vi "DropDown VI Wrapper.vi"(7 "Software Config File Path":path) -> ()   [LabVIEW 2016]
uses:
  DropDown VI Wrapper Type Defs/Drop Down Control.ctl
  <vilib>/Utility/miscctls.llb/LVPointTypeDef.ctl
  <vilib>/Utility/miscctls.llb/LVRectTypeDef.ctl
panel:
  in  "Screen and Exit Bar":T1
  in  "Drop Down Control 1":T2
  in  "Drop Down Control 2":T2
  in  "Drop Down Control 3":T2
  in  "Drop Down Control 4":T2
  in  "Drop Down Control 5":T2
  in  "Drop Down Control 6":T2
  in  "Drop Down Control 7":T2
  in  "Drop Down Control 8":T2
  in  "Drop Down Control 9":T2
  in  "Drop Down Control 10":T2
  # "Device Panel"
  # "Laser Control"
  # "XY Control"
  # "Camera Control"
  # "Blank 01"
  # "Blank 01"
  # "Name Here"
  # "Name Here"
  # "Name Here"
  # "Name Here"
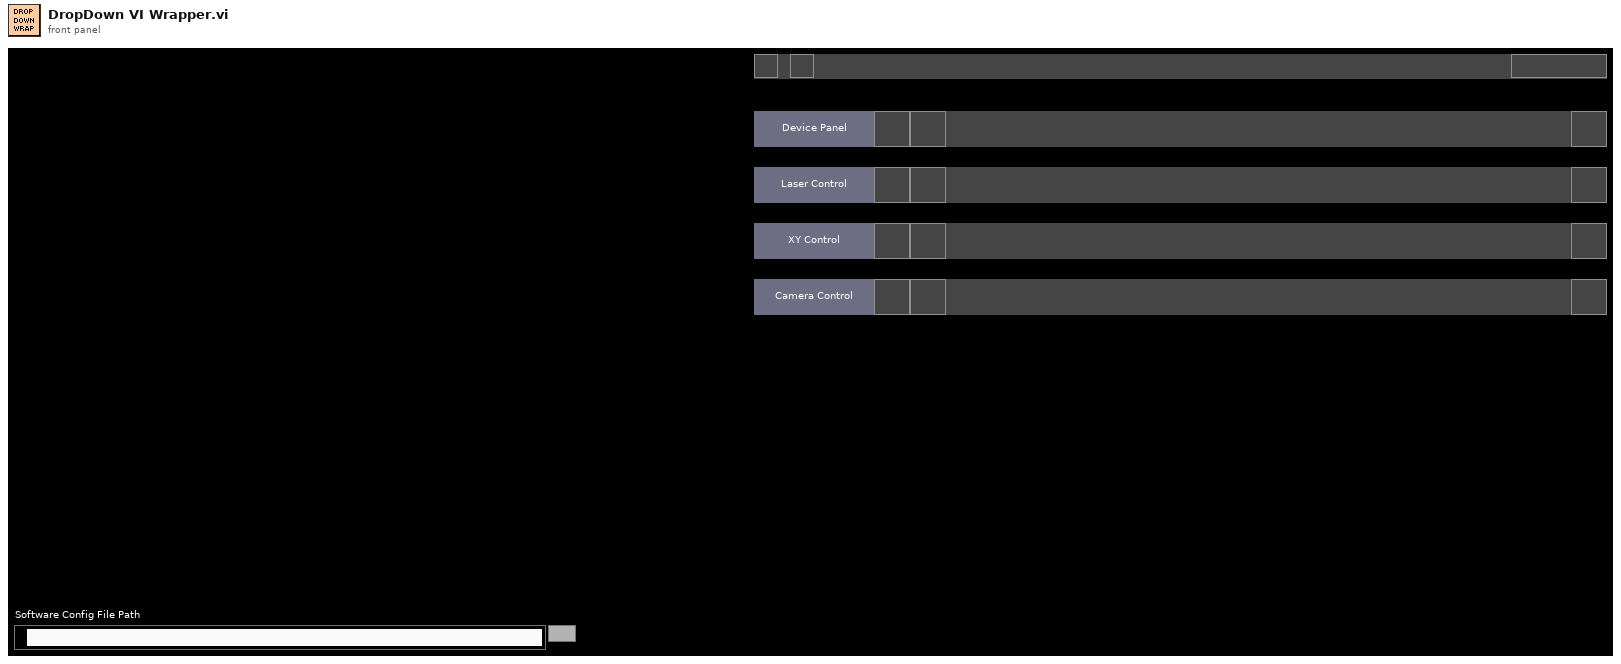
[diagram p1: front panel]
types:
  T1 = cluster{"Max Left":bool, "Max Right":bool, "Exit":bool, "Messages":string}
  T2 = typedef "Drop Down Control.ctl" = cluster{"Right Width":bool, "Messages":string, "Abort VI":bool, "Close VI":bool}
  T3 = enum16{"Always On", "Always Off", "Off While Running"}
  T4 = typedef "LVPointTypeDef.ctl" = cluster{"Horizontal":i16, "Vertical":i16}
  T5 = enum32{"Invalid", "Standard", "Closed", "Hidden", "Minimized", "Maximized"}
  T6 = typedef "LVRectTypeDef.ctl" = cluster{"Left":i16, "Top":i16, "Right":i16, "Bottom":i16}
  T7 = enum8{"Enabled", "Disabled", "Disabled and Grayed Out"}
  T8 = cluster{"VI Path":path, "VI Refnum":refnum<vi>}[]
  T9 = typedef "lveventtype.ctl" = enum32{"Null", "Timeout", "Annotation Menu Selection", "Annotation Menu Selection?", "App Instance Close", "App Instance Close?", "Autoscale Range Change", "Bookmark Info Change", "Cell Edit", "Cell Edit?", "Cursor Grab", "Cursor Grab?", "Cursor Menu Selection", "Cursor Menu Selection?", "Cursor Move", "Cursor Release", "Data Change", "Direction Change", "Display State Change", "Drag Ended", "Drag Enter", "Drag Leave", "Drag Over", "Drag Source Update", "Drag Starting", "Drag Starting?", "Drop", "Exec State Change", "Key Down", "Key Down?", "Key Repeat", "Key Repeat?", "Key Up", "Listbox Double Click", "Menu Activation?", "Menu Selection (App)", "Menu Selection? (App)", "Menu Selection (User)", "Mouse Down", "Mouse Down?", "Mouse Enter", "Mouse Leave", "Mouse Move", "Mouse Up", "Mouse Wheel", "NI Security User Change (App)", "Pane Size", "Panel Close", "Panel Close?", "Panel Resize", "Plot Attribute Change", "Scale Range Change", "Shortcut Menu Activation?", "Shortcut Menu Selection (App)", "Shortcut Menu Selection? (App)", "Shortcut Menu Selection (User)", "Tree Double Click", "Tree Drag", "Tree Drag?", "Tree Drop", "Tree Drop?", "Tree Item Close", "Tree Item Close?", "Tree Item Open", "Tree Item Open?", "User Event", "Value Change"}
  T10 = typedef "LVAllMonitorsDisplayTypeDef.ctl" = cluster{"Bounds":cluster{"Left":i16, "Top":i16, "Right":i16, "Bottom":i16}, "Depth":i16}[]
  T11 = cluster{"Bounds":cluster{"Left":i16, "Top":i16, "Right":i16, "Bottom":i16}, "Depth":i16}
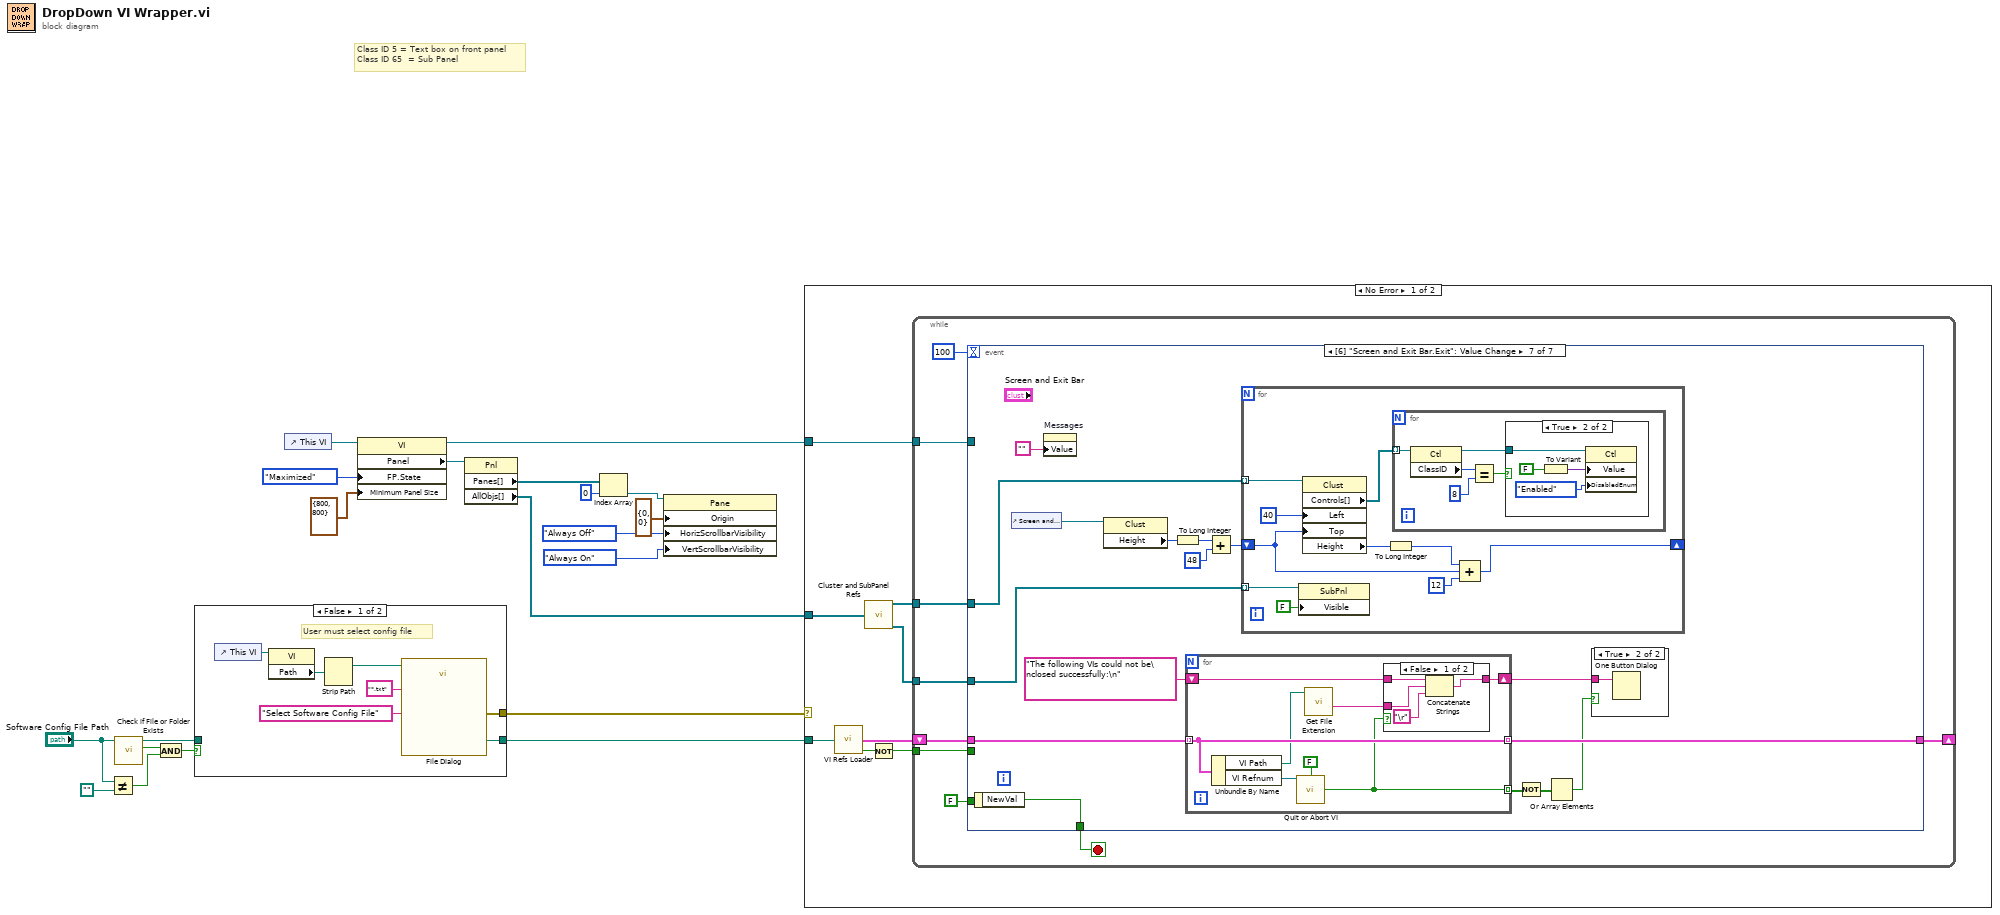
[diagram p0: block diagram]
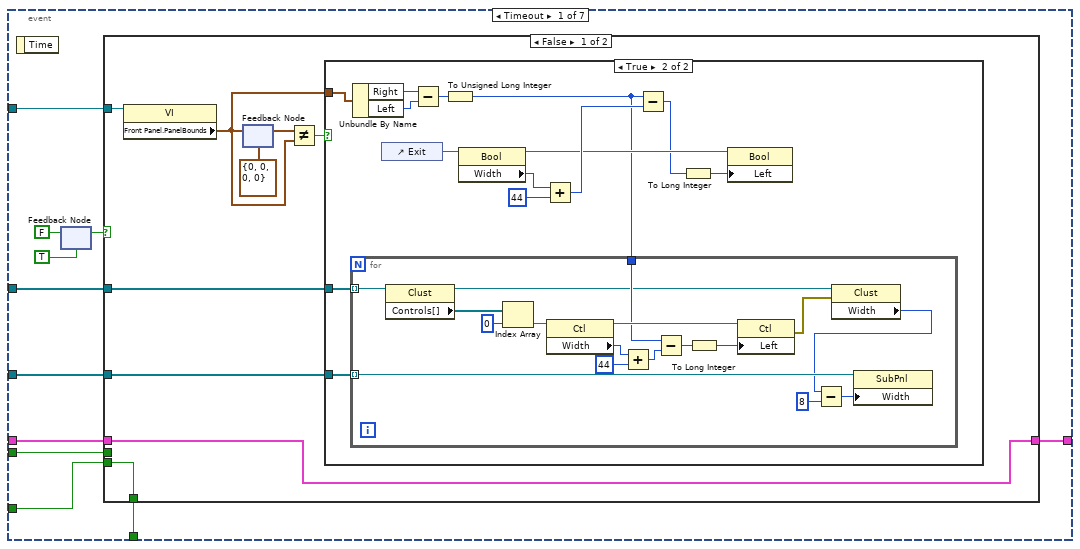
[diagram p2: hidden frame]
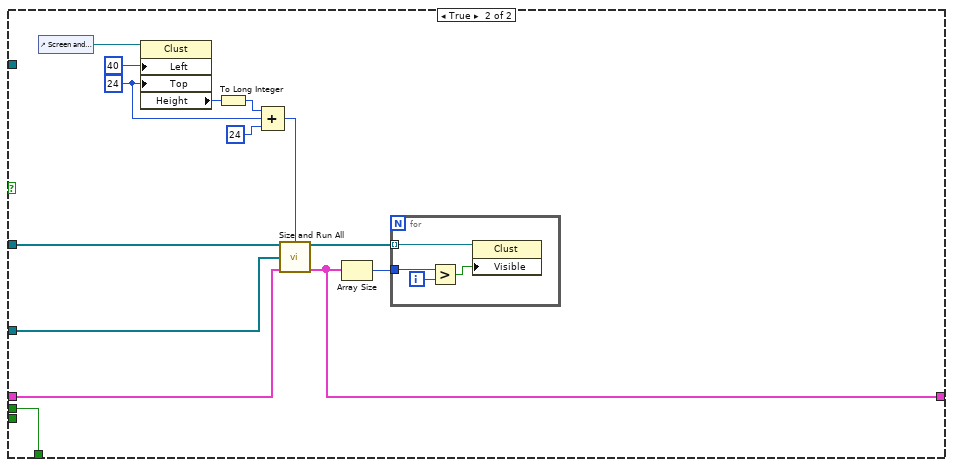
[diagram p4: hidden frame]
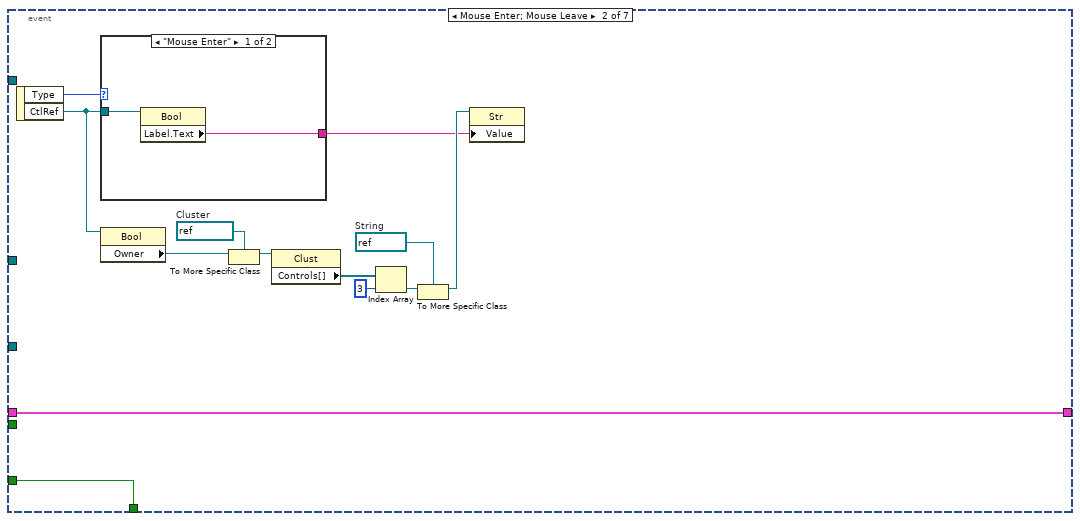
[diagram p5: hidden frame]
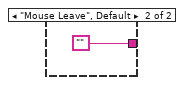
[diagram p6: hidden frame]
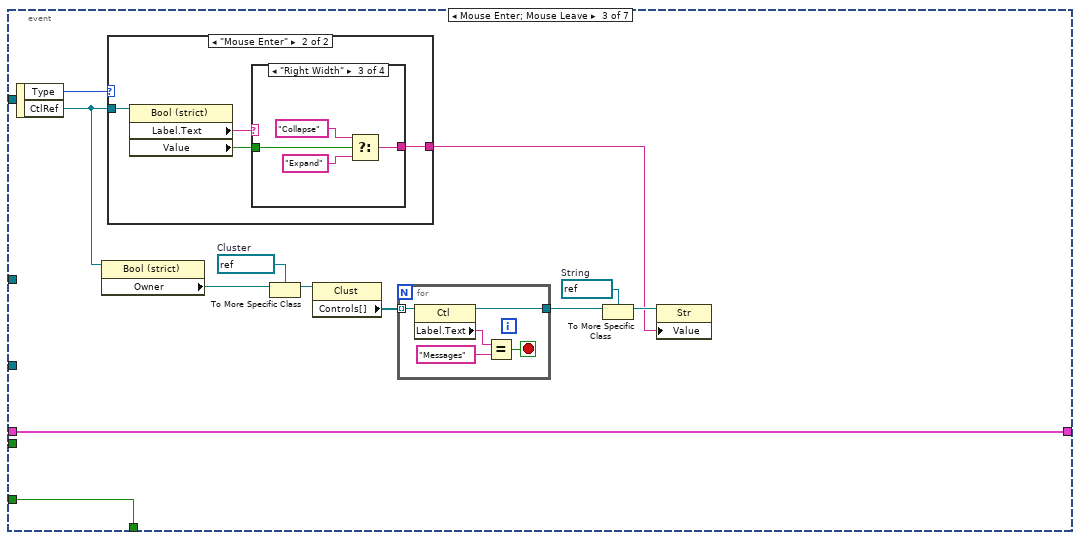
[diagram p7: hidden frame]
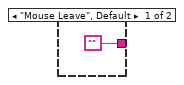
[diagram p8: hidden frame]
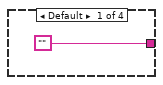
[diagram p9: hidden frame]
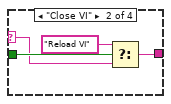
[diagram p10: hidden frame]
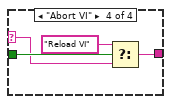
[diagram p11: hidden frame]
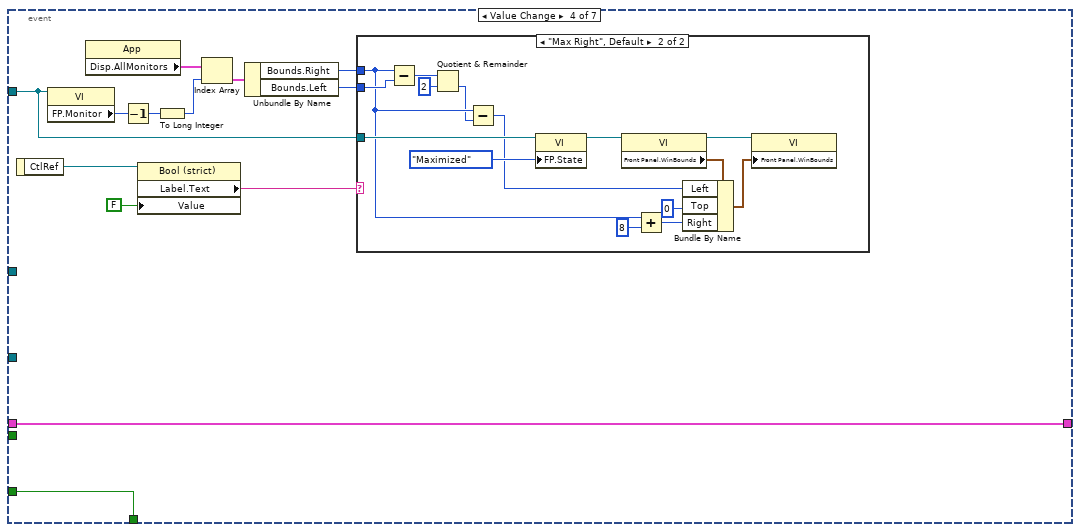
[diagram p12: hidden frame]
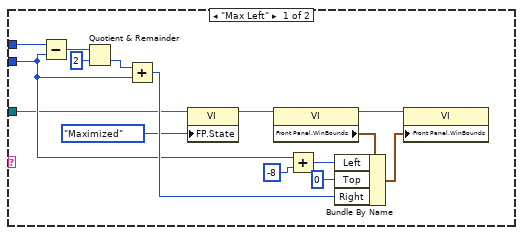
[diagram p13: hidden frame]
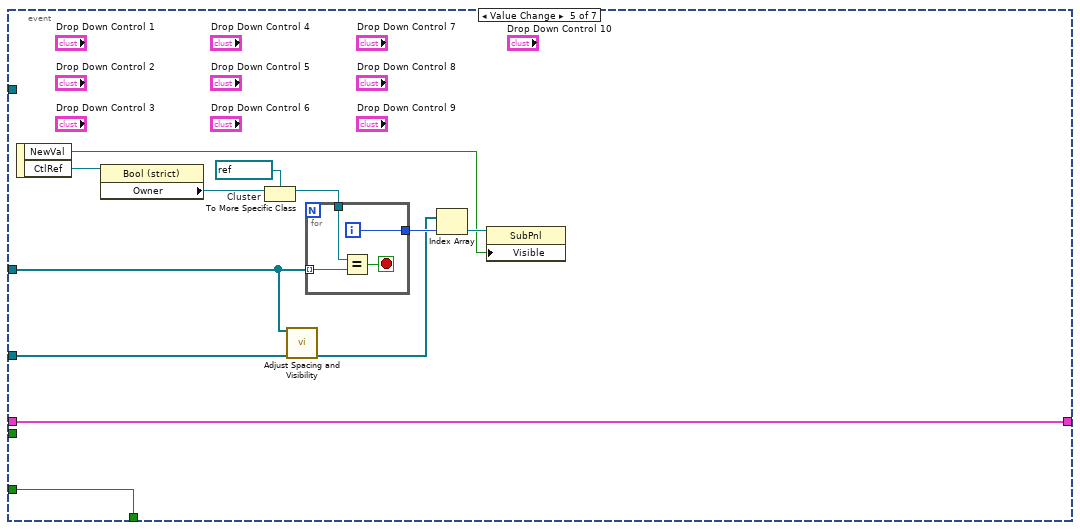
[diagram p14: hidden frame]
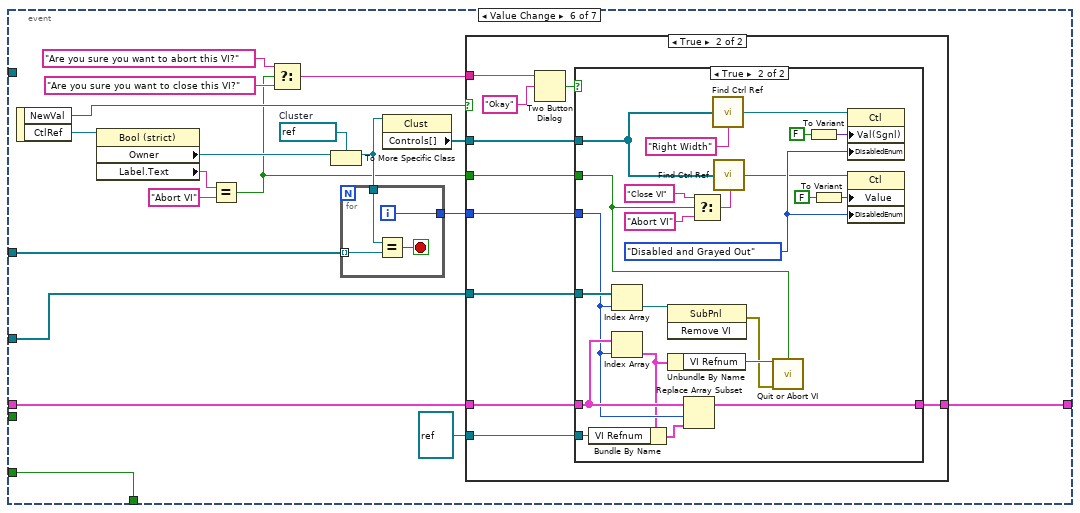
[diagram p15: hidden frame]
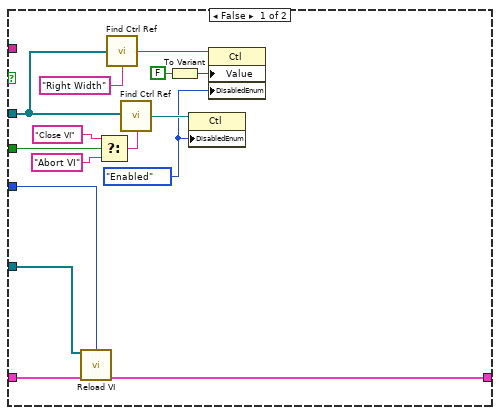
[diagram p16: hidden frame]
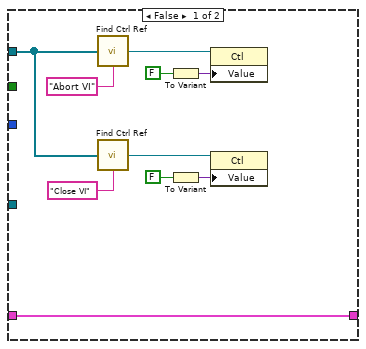
[diagram p17: hidden frame]
diagram:
  # "Class ID 5 = Text box on front panel\nClass ID 65  = Sub Panel"
  n1 = Not Equal?(x="Software Config File Path", y=path "") -> (x != y?=w7:bool)
  n2 = call <vilib>:"Check if File or Folder Exists.vi"("path"="Software Config File Path") -> ("file or folder exists?"=w6:bool, "dup path"=w4:path)  [unwired: 8 in, 1 out]
  n3 = And(x=w6, y=w7) -> (x .and. y?=w5:bool)
  n4 = case shown="False" w5 {
    tunnel: w4 -> [_ w29]
    tunnel: [w25 w29] -> w1
    tunnel: [w24 errorcluster {"status"=FALSE, "code"=0, "source"=""} ("error out")] -> w2
    frame False {
      # "User must select config file"
      n5 = control-ref of="This VI"() -> (w23:refnum<vi>)
      n6 = property class="VI"(reference=w23) -> ("Path"=w22:path)  [unwired: 1 in, 2 out]
      n7 = Strip Path(path=w22) -> (stripped path=w21:path)  [unwired: 1 out]
      n8 = call "File Dialog"("start path"=w21, "prompt"="Select Software Config File", "pattern (all files)"="*.txt") -> ("selected path"=w25:path, "error out"=w24:errorcluster)  [unwired: 9 in, 2 out]
    }
    frame True {
      # "Config File is specified - try and use it"
    }
  }
  n9 = control-ref of="This VI"() -> (w16:refnum<vi>)
  n10 = property class="VI"(reference=w16, "FP.State"=T5."Maximized" ("Front Panel Window:State"), "Minimum Panel Size"=T4 {"Horizontal"=800, "Vertical"=800} ("Front Panel Window:Minimum Size")) -> (reference out=w11:refnum<vi>, "Panel"=w10:refnum<vi>)  [unwired: 1 in, 1 out]
  n11 = property class="Pnl"(reference=w10) -> ("Panes[]"=w13:refnum<vi>[], "AllObjs[]"=w9:refnum<vi>[])  [unwired: 1 in, 2 out]
  n12 = Index Array(array=w13, index=0) -> (element=w19:refnum<vi>)
  n13 = property class="Pane"(reference=w19, "Origin"=T4 {"Horizontal"=0, "Vertical"=0}, "HorizScrollbarVisibility"=T3."Always Off" ("Vertical Scrollbar Visibility"), "VertScrollbarVisibility"=T3."Always On" ("Vertical Scrollbar Visibility")) -> ()  [unwired: 1 in, 2 out]
  n14 = case shown="No Error" w2 {
    tunnel: w11 -> [w37 _]
    tunnel: w9 -> [w33 _]
    tunnel: w1 -> [w30 _]
    frame No Error {
      n15 = call "VI Refs Loader.vi"("Config File Path"=w30) -> ("VI Path/Ref"=w32:T8, "VIs Loaded?"=w36:bool)  [unwired: 12 in, 1 out]
      n16 = call "Cluster and SubPanel Refs.vi"("All Objects Refs"=w33) -> ("Cluster Refs"=w35:refnum<vi>[], "Sub Panel Refs"=w34:refnum<vi>[])  [unwired: 13 in]
      n17 = Not(x=w36) -> (.not. x?=w31:bool)
      n18 = while {
        tunnel: w37 -> [w43]
        tunnel: w35 -> [w38]
        tunnel: w34 -> [w41]
        tunnel: w31 -> [w40]
        shift-right: [w39] -> _
        shift-left: w32 -> [w42]
        stop <- w46 stop-if-true
        n19 = event shown="[6] \"Screen and Exit Bar.Exit\": Value Change" {
          selector: _ -> [_ _ _ _ _ _ _]
          dyn-events: _ -> [_ _ _ _ _ _ _]
          timeout: 100 -> [_ _ _ _ _ _ _]
          tunnel: [w53 w128 w142 w179 w221 w244 w322] -> w46
          tunnel: FALSE -> [w52 w128 w142 w179 w221 w244 _]
          tunnel: w43 -> [w57 _ _ w170 _ _ _]
          tunnel: w38 -> [w56 _ _ _ w215 w239 w320]
          tunnel: w41 -> [w55 _ _ _ w216 w237 w319]
          tunnel: w42 -> [w54 w116 w143 w167 w210 w238 w313]
          tunnel: w40 -> [w51 _ _ _ _ _ _]
          tunnel: [w50 w116 w143 w167 w210 w235 w312] -> w39
          event Timeout {
            n20 = event-data() -> ()  [unwired: 1 in, 1 out]
            n21 = feedback #1(TRUE) -> (w47:bool)
            n22 = feedback-in #1(FALSE) -> ()
            n23 = case shown="False" w47 {
              tunnel: w57 -> [w66 _]
              tunnel: w56 -> [w61 w102]
              tunnel: w55 -> [w60 w109]
              tunnel: w54 -> [w58 w108]
              tunnel: [w59 w99] -> w53
              tunnel: w52 -> [w59 _]
              tunnel: w51 -> [_ w99]
              tunnel: [w58 w98] -> w50
              frame False {
                n24 = property class="VI"(reference=w66) -> ("Front Panel.PanelBounds"=w62:T6)  [unwired: 1 in, 2 out]
                n25 = feedback-in #2(w62) -> ()
                n26 = feedback #2(T6 {"Left"=0, "Top"=0, "Right"=0, "Bottom"=0} ("Front Panel.PanelBounds")) -> (w65:T6)
                n27 = Not Equal?(x=w65, y=w62) -> (x != y?=w63:bool)
                n28 = case shown="True" w63 {
                  tunnel: w62 -> [_ w80]
                  tunnel: w61 -> [_ w70]
                  tunnel: w60 -> [_ w67]
                  frame False {
                  }
                  frame True {
                    n29 = Unbundle By Name(w80) -> ("Right"=w72:i16, "Left"=w73:i16)
                    n30 = control-ref of="Exit"() -> (w78:refnum<vi>)
                    n31 = Subtract(x=w72, y=w73) -> (x-y=w71:i16)
                    n32 = To Unsigned Long Integer(number=w71) -> (unsigned 32bit integer=w68:u32)
                    n33 = for {
                      tunnel: w70 -> [w97] mode=indexing
                      tunnel: w68 -> [w88]
                      tunnel: w67 -> [w86] mode=indexing
                      n34 = property class="Clust"(reference=w97) -> (reference out=w85:refnum<vi>, "Controls[]"=w96:refnum<vi>[])  [unwired: 1 in, 1 out]
                      n35 = Index Array(array=w96, index=0) -> (element=w92:refnum<vi>)
                      n36 = property class="Ctl"(reference=w92) -> (reference out=w91:refnum<vi>, "Width"=w93:u32)  [unwired: 1 in, 1 out]
                      n37 = Add(x=w93, y=u32 44) -> (x+y=w90:u32)
                      n38 = Subtract(x=w88, y=w90) -> (x-y=w89:u32)
                      n39 = To Long Integer(number=w89) -> (32bit integer=w94:i32)
                      n40 = property class="Ctl"(reference=w91, "Left"=w94) -> (error out=w84:errorcluster)  [unwired: 1 in, 1 out]
                      n41 = property class="Clust"(reference=w85, error in=w84) -> ("Width"=w83:u32)  [unwired: 2 out]
                      n42 = Subtract(x=w83, y=u32 8) -> (x-y=w82:u32)
                      n43 = property class="SubPnl"(reference=w86, "Width"=w82) -> ()  [unwired: 1 in, 2 out]
                    }
                    n44 = property class="Bool"(reference=w78) -> (reference out=w76:refnum<vi>, "Width"=w79:u32)  [unwired: 1 in, 1 out]
                    n45 = Add(x=w79, y=u32 44) -> (x+y=w77:u32)
                    n46 = Subtract(x=w68, y=w77) -> (x-y=w74:u32)
                    n47 = To Long Integer(number=w74) -> (32bit integer=w75:i32)
                    n48 = property class="Bool"(reference=w76, "Left"=w75) -> ()  [unwired: 1 in, 2 out]
                  }
                }
              }
              frame True {
                w106 = 24 ("Position:Top")
                n49 = control-ref of="Screen and Exit Bar"() -> (w111:refnum<vi>)
                n50 = property class="Clust"(reference=w111, "Left"=40 ("Position:Left"), "Top"=w106) -> ("Height"=w107:u32)  [unwired: 1 in, 2 out]
                n51 = To Long Integer(number=w107) -> (32bit integer=w105:i32)
                n52 = Compound Arithmetic op=ADD(w105, w106, 24 ("value")) -> (w103:i32)
                n53 = call "Size and Run All.vi"("Cluster Refs"=w102, "Initial Top Position"=w103, "Subpanel Refs"=w109, "VI Path/Ref"=w108) -> ("Cluster Refs Dup"=w101:refnum<vi>[], "VI Path/Ref Out"=w98:T8)  [unwired: 10 in]
                n54 = Array Size(array=w98) -> (size(s)=w100:i32)
                n55 = for {
                  tunnel: w101 -> [w115] mode=indexing
                  tunnel: w100 -> [w112]
                  i -> [w114]
                  n56 = Greater?(x=w112, y=w114) -> (0:w113:bool)
                  n57 = property class="Clust"(reference=w115, "Visible"=w113) -> ()  [unwired: 1 in, 2 out]
                }
              }
            }
          }
          event "Screen and Exit Bar.Exit", "Screen and Exit Bar.Max Right", "Screen and Exit Bar.Max Left": Mouse Enter; "Screen and Exit Bar.Exit", "Screen and Exit Bar.Max Right", "Screen and Exit Bar.Max Left": Mouse Leave {
            w119 = refnum<vi> refnum  # String
            w124 = refnum<vi> refnum  # Cluster
            n58 = event-data() -> ("Type"=w127:T9, "CtlRef"=w126:refnum<vi>)  [unwired: 1 in]
            n59 = case shown="\"Mouse Enter\"" w127 {
              tunnel: w126 -> [w130 _]
              tunnel: [w129 ""] -> w117
              frame "Mouse Enter" {
                n60 = property class="Bool"(reference=w130) -> ("Label.Text"=w129:string)  [unwired: 1 in, 2 out]
              }
              frame "Mouse Leave", Default {
              }
            }
            n61 = property class="Bool"(reference=w126) -> ("Owner"=w125:refnum<vi>)  [unwired: 1 in, 2 out]
            n62 = To More Specific Class(target class=w124, reference=w125) -> (specific class reference=w123:refnum<vi>)  [unwired: 1 in, 1 out]
            n63 = property class="Clust"(reference=w123) -> ("Controls[]"=w122:refnum<vi>[])  [unwired: 1 in, 2 out]
            n64 = Index Array(array=w122, index=3) -> (element=w120:refnum<vi>)
            n65 = To More Specific Class(target class=w119, reference=w120) -> (specific class reference=w118:refnum<vi>)  [unwired: 1 in, 1 out]
            n66 = property class="Str"(reference=w118, "Value"=w117) -> ()  [unwired: 1 in, 2 out]
          }
          event Mouse Enter; Mouse Leave {
            w134 = refnum<vi> refnum  # String
            w139 = refnum<vi> refnum  # Cluster
            n67 = event-data() -> ("Type"=w141:T9, "CtlRef"=w140:refnum<vi>)  [unwired: 1 in]
            n68 = property class="Bool (strict)"(reference=w140) -> ("Owner"=w137:refnum<vi>)  [unwired: 1 in, 2 out]
            n69 = case shown="\"Mouse Enter\"" w141 {
              tunnel: w140 -> [_ w153]
              tunnel: ["" w150] -> w132
              frame "Mouse Leave", Default {
              }
              frame "Mouse Enter" {
                n70 = property class="Bool (strict)"(reference=w153) -> ("Label.Text"=w152:string, "Value"=w151:bool)  [unwired: 1 in, 2 out]
                n71 = case shown="\"Right Width\"" w152 {
                  selector: w152 -> [_ w157 _ w164]
                  tunnel: w151 -> [_ w158 w162 w165]
                  tunnel: ["" w155 w159 w163] -> w150
                  frame Default {
                  }
                  frame "Close VI" {
                    n72 = Select(t="Reload VI", s=w158, f=w157) -> (s? t:f=w155:string)
                  }
                  frame "Right Width" {
                    n73 = Select(t="Collapse", s=w162, f="Expand") -> (s? t:f=w159:string)
                  }
                  frame "Abort VI" {
                    n74 = Select(t="Reload VI", s=w165, f=w164) -> (s? t:f=w163:string)
                  }
                }
              }
            }
            n75 = To More Specific Class(target class=w139, reference=w137) -> (specific class reference=w138:refnum<vi>)  [unwired: 1 in, 1 out]
            n76 = property class="Clust"(reference=w138) -> ("Controls[]"=w136:refnum<vi>[])  [unwired: 1 in, 2 out]
            n77 = for {
              tunnel: w136 -> [w148] mode=indexing
              tunnel: [w144] -> w135
              stop <- w145 stop-if-true
              n78 = property class="Ctl"(reference=w148) -> (reference out=w144:refnum<vi>, "Label.Text"=w147:string)  [unwired: 1 in, 1 out]
              n79 = Equal?(x=w147, y="Messages") -> (x = y?=w145:bool)
            }
            n80 = To More Specific Class(target class=w134, reference=w135) -> (specific class reference=w133:refnum<vi>)  [unwired: 1 in, 1 out]
            n81 = property class="Str"(reference=w133, "Value"=w132) -> ()  [unwired: 1 in, 2 out]
          }
          event "Screen and Exit Bar.Max Right", "Screen and Exit Bar.Max Left": Value Change {
            n82 = event-data() -> ("CtlRef"=w178:refnum<vi>)  [unwired: 1 in]
            n83 = property class="VI"(reference=w170) -> ("FP.Monitor"=w177:u16)  [unwired: 1 in, 2 out]
            n84 = property class="App"() -> ("Disp.AllMonitors"=w176:T10)  [unwired: 2 in, 2 out]
            n85 = Decrement(x=w177) -> (x-1=w175:u16)
            n86 = property class="Bool (strict)"(reference=w178, "Value"=FALSE) -> ("Label.Text"=w169:string)  [unwired: 1 in, 2 out]
            n87 = To Long Integer(number=w175) -> (32bit integer=w174:i32)
            n88 = Index Array(array=w176, index=w174) -> (element=w173:T11)
            n89 = Unbundle By Name(w173) -> ("Bounds.Right"=w172:i16, "Bounds.Left"=w171:i16)
            n90 = case shown="\"Max Right\", Default" w169 {
              tunnel: w172 -> [w194 w197]
              tunnel: w171 -> [w182 w201]
              tunnel: w170 -> [w180 w200]
              frame "Max Left" {
                n91 = Subtract(x=w194, y=w182) -> (x-y=w189:i16)
                n92 = Quotient & Remainder(x=w189, y=i16 2) -> (floor(x/y)=w187:i16)  [unwired: 1 out]
                n93 = Add(x=w187, y=w182) -> (x+y=w186:i16)
                n94 = property class="VI"(reference=w180, "FP.State"=T5."Maximized" ("Front Panel Window:State")) -> (reference out=w184:refnum<vi>)  [unwired: 1 in, 1 out]
                n95 = property class="VI"(reference=w184) -> (reference out=w193:refnum<vi>, "Front Panel.WinBounds"=w191:T6)  [unwired: 1 in, 1 out]
                n96 = Add(x=w182, y=i16 -8 ("Left")) -> (x+y=w181:i16)
                n97 = Bundle By Name(cluster=w191, "Left"=w181, "Top"=i16 0, "Right"=w186) -> (w192:T6)
                n98 = property class="VI"(reference=w193, "Front Panel.WinBounds"=w192) -> ()  [unwired: 1 in, 2 out]
              }
              frame "Max Right", Default {
                n99 = Subtract(x=w197, y=w201) -> (x-y=w206:i16)
                n100 = Quotient & Remainder(x=w206, y=i16 2) -> (floor(x/y)=w196:i16)  [unwired: 1 out]
                n101 = Subtract(x=w197, y=w196) -> (x-y=w195:i16)
                n102 = property class="VI"(reference=w200, "FP.State"=T5."Maximized" ("Front Panel Window:State")) -> (reference out=w203:refnum<vi>)  [unwired: 1 in, 1 out]
                n103 = property class="VI"(reference=w203) -> (reference out=w209:refnum<vi>, "Front Panel.WinBounds"=w207:T6)  [unwired: 1 in, 1 out]
                n104 = Add(x=w197, y=i16 8 ("Left")) -> (x+y=w198:i16)
                n105 = Bundle By Name(cluster=w207, "Left"=w195, "Top"=i16 0, "Right"=w198) -> (w208:T6)
                n106 = property class="VI"(reference=w209, "Front Panel.WinBounds"=w208) -> ()  [unwired: 1 in, 2 out]
              }
            }
          }
          event Value Change {
            w212 = refnum<vi> refnum  # Cluster
            n107 = event-data() -> ("NewVal"=w217:bool, "CtlRef"=w214:refnum<vi>)  [unwired: 1 in]
            n108 = property class="Bool (strict)"(reference=w214) -> ("Owner"=w213:refnum<vi>)  [unwired: 1 in, 2 out]
            n109 = To More Specific Class(target class=w212, reference=w213) -> (specific class reference=w211:refnum<vi>)  [unwired: 1 in, 1 out]
            n110 = call "Adjust Spacing and Visibility.vi"("Cluster Ref Array"=w215, "Sub Panel Ref Array"=w216) -> ("Sub Panel Ref Array Dup"=w219:refnum<vi>[])  [unwired: 13 in]
            n111 = for {
              tunnel: w215 -> [w225] mode=indexing
              tunnel: w211 -> [w224]
              tunnel: [w222] -> w220
              i -> [w222]
              stop <- w223 stop-if-true
              n112 = Equal?(x=w224, y=w225) -> (x = y?=w223:bool)
            }
            n113 = Index Array(array=w219, index=w220) -> (element=w218:refnum<vi>)
            n114 = property class="SubPnl"(reference=w218, "Visible"=w217) -> ()  [unwired: 1 in, 2 out]
          }
          event Value Change {
            w242 = refnum<vi> refnum  # Cluster
            n115 = event-data() -> ("NewVal"=w236:bool, "CtlRef"=w241:refnum<vi>)  [unwired: 1 in]
            n116 = property class="Bool (strict)"(reference=w241) -> ("Owner"=w243:refnum<vi>, "Label.Text"=w233:string)  [unwired: 1 in, 2 out]
            n117 = Equal?(x=w233, y="Abort VI" ("message")) -> (x = y?=w226:bool)
            n118 = Select(t="Are you sure you want to abort this VI?" ("message"), s=w226, f="Are you sure you want to close this VI?" ("message")) -> (s? t:f=w229:string)
            n119 = To More Specific Class(target class=w242, reference=w243) -> (specific class reference=w228:refnum<vi>)  [unwired: 1 in, 1 out]
            n120 = for {
              tunnel: w239 -> [w306] mode=indexing
              tunnel: w228 -> [w305]
              tunnel: [w303] -> w240
              i -> [w303]
              stop <- w304 stop-if-true
              n121 = Equal?(x=w305, y=w306) -> (x = y?=w304:bool)
            }
            n122 = property class="Clust"(reference=w228) -> ("Controls[]"=w227:refnum<vi>[])  [unwired: 1 in, 2 out]
            n123 = case shown="True" w236 {
              tunnel: w240 -> [w256 w267]
              tunnel: w238 -> [w258 w266]
              tunnel: w237 -> [w259 w265]
              tunnel: w227 -> [w246 w261]
              tunnel: [w257 w264] -> w235
              tunnel: refnum<vi> refnum ("VI Refnum") -> [_ w263]
              tunnel: w229 -> [_ w262]
              tunnel: w226 -> [w252 w260]
              frame False {
                w245 = T7."Enabled" ("Disabled")
                n124 = call "Reload VI.vi"("Sub Panel Refs"=w259, "Index"=w256, "Path/Ref Array In"=w258) -> ("Updated Path/Ref Array"=w257:T8)  [unwired: 12 in]
                n125 = Select(t="Close VI" ("message"), s=w252, f="Abort VI" ("message")) -> (s? t:f=w253:string)
                n126 = call "Find Ctrl Ref.vi"("Control Array"=w246, "Control Label"="Right Width") -> ("Control Ref"=w249:refnum<vi>)  [unwired: 12 in, 1 out]
                n127 = call "Find Ctrl Ref.vi"("Control Array"=w246, "Control Label"=w253) -> ("Control Ref"=w251:refnum<vi>)  [unwired: 12 in, 1 out]
                n128 = To Variant(anything=FALSE) -> (Variant=w247:variant)
                n129 = property class="Ctl"(reference=w251, "DisabledEnum"=w245) -> ()  [unwired: 1 in, 2 out]
                n130 = property class="Ctl"(reference=w249, "Value"=w247, "DisabledEnum"=w245) -> ()  [unwired: 1 in, 2 out]
              }
              frame True {
                n131 = Two Button Dialog(message=w262, 2:"Okay" ("T button name (\"OK\")")) -> (T button?=w268:bool)  [unwired: 1 in]
                n132 = case shown="True" w268 {
                  tunnel: w267 -> [_ w297]
                  tunnel: w265 -> [_ w302]
                  tunnel: w266 -> [w279 w298]
                  tunnel: [w279 w295] -> w264
                  tunnel: w263 -> [_ w294]
                  tunnel: w261 -> [w273 w285]
                  tunnel: w260 -> [_ w287]
                  frame False {
                    n133 = call "Find Ctrl Ref.vi"("Control Array"=w273, "Control Label"="Abort VI") -> ("Control Ref"=w274:refnum<vi>)  [unwired: 12 in, 1 out]
                    n134 = call "Find Ctrl Ref.vi"("Control Array"=w273, "Control Label"="Close VI") -> ("Control Ref"=w272:refnum<vi>)  [unwired: 12 in, 1 out]
                    n135 = To Variant(anything=FALSE) -> (Variant=w277:variant)
                    n136 = To Variant(anything=FALSE) -> (Variant=w276:variant)
                    n137 = property class="Ctl"(reference=w274, "Value"=w277) -> ()  [unwired: 1 in, 2 out]
                    n138 = property class="Ctl"(reference=w272, "Value"=w276) -> ()  [unwired: 1 in, 2 out]
                  }
                  frame True {
                    w283 = T7."Disabled and Grayed Out" ("Disabled")
                    n139 = Index Array(array=w302, index=w297) -> (element=w301:refnum<vi>)
                    n140 = Index Array(array=w298, index=w297) -> (element=w293:cluster{"VI Path":path, "VI Refnum":refnum<vi>})
                    n141 = Bundle By Name(cluster=w293, "VI Refnum"=w294) -> (w296:cluster{"VI Path":path, "VI Refnum":refnum<vi>})
                    n142 = invoke class="SubPnl" method="Remove VI"(reference=w301) -> (error out=w288:errorcluster)  [unwired: 2 in, 2 out]
                    n143 = Unbundle By Name(w293) -> ("VI Refnum"=w289:refnum<vi>)
                    n144 = Replace Array Subset(array=w298, new element=w296, index=w297) -> (w295:T8)
                    n145 = Select(t="Close VI" ("message"), s=w287, f="Abort VI" ("message")) -> (s? t:f=w290:string)
                    n146 = call "Find Ctrl Ref.vi"("Control Array"=w285, "Control Label"="Right Width") -> ("Control Ref"=w284:refnum<vi>)  [unwired: 12 in, 1 out]
                    n147 = call "Find Ctrl Ref.vi"("Control Array"=w285, "Control Label"=w290) -> ("Control Ref"=w280:refnum<vi>)  [unwired: 12 in, 1 out]
                    n148 = call "Quit or Abort VI.vi"("VI Ref"=w289, "Abort VI?"=w287, "Error In"=w288) -> ()  [unwired: 12 in, 1 out]
                    n149 = To Variant(anything=FALSE) -> (Variant=w281:variant)
                    n150 = To Variant(anything=FALSE) -> (Variant=w300:variant)
                    n151 = property class="Ctl"(reference=w284, "Val(Sgnl)"=w281, "DisabledEnum"=w283) -> ()  [unwired: 1 in, 2 out]
                    n152 = property class="Ctl"(reference=w280, "Value"=w300, "DisabledEnum"=w283) -> ()  [unwired: 1 in, 2 out]
                  }
                }
              }
            }
          }
          event "Screen and Exit Bar.Exit": Value Change {
            n153 = event-data() -> ("NewVal"=w322:bool)  [unwired: 1 in]
            n154 = control-ref of="Screen and Exit Bar"() -> (w316:refnum<vi>)
            n155 = property on="Messages" class="Str"("Value"="") -> ()  [unwired: 2 in, 2 out]
            n156 = property class="Clust"(reference=w316) -> ("Height"=w315:u32)  [unwired: 1 in, 2 out]
            n157 = To Long Integer(number=w315) -> (32bit integer=w317:i32)
            n158 = for {
              tunnel: w313 -> [w331] mode=indexing
              tunnel: [w331] -> w312 mode=indexing
              shift-right: [w325] -> w307
              shift-left: "The following VIs could not be\nclosed successfully:\n" -> [w326]
              tunnel: [w324] -> w310 mode=indexing
              n159 = Unbundle By Name(w331) -> ("VI Path"=w328:path, "VI Refnum"=w330:refnum<vi>)
              n160 = call "Quit or Abort VI.vi"("VI Ref"=w330, "Abort VI?"=FALSE) -> ("Close Command Successful?"=w324:bool)  [unwired: 13 in]
              n161 = call <vilib>:"Get File Extension.vi"("file"=w328) -> ("filename without extension"=w327:string)  [unwired: 6 in, 4 out]
              n162 = case shown="False" w324 {
                tunnel: w327 -> [w334 _]
                tunnel: w326 -> [w333 w336]
                tunnel: [w332 w336] -> w325
                frame False {
                  n163 = Concatenate Strings(w333, w334, "\r") -> (w332:string)
                }
                frame True {
                }
              }
            }
            n164 = Add(x=w317, y=48) -> (x+y=w314:i32)
            n165 = for {
              tunnel: w320 -> [w345] mode=indexing
              shift-right: [w344] -> _
              shift-left: w314 -> [w340]
              tunnel: w319 -> [w337] mode=indexing
              n166 = property class="SubPnl"(reference=w337, "Visible"=FALSE) -> ()  [unwired: 1 in, 2 out]
              n167 = property class="Clust"(reference=w345, "Left"=40 ("Position:Left"), "Top"=w340) -> ("Controls[]"=w339:refnum<vi>[], "Height"=w342:u32)  [unwired: 1 in, 2 out]
              n168 = To Long Integer(number=w342) -> (32bit integer=w341:i32)
              n169 = for {
                tunnel: w339 -> [w351] mode=indexing
                n170 = property class="Ctl"(reference=w351) -> (reference out=w347:refnum<vi>, "ClassID"=w350:u32)  [unwired: 1 in, 1 out]
                n171 = Equal?(x=w350, y=u32 8) -> (x = y?=w348:bool)
                n172 = case shown="True" w348 {
                  tunnel: w347 -> [_ w353]
                  frame False {
                  }
                  frame True {
                    n173 = To Variant(anything=FALSE) -> (Variant=w354:variant)
                    n174 = property class="Ctl"(reference=w353, "Value"=w354, "DisabledEnum"=T7."Enabled" ("Disabled")) -> ()  [unwired: 1 in, 2 out]
                  }
                }
              }
              n175 = Compound Arithmetic op=ADD(w341, w340, 12 ("value")) -> (w344:i32)
            }
            n176 = Not(x=w310) -> (.not. x?=w309:bool[])
            n177 = Or Array Elements(Boolean array=w309) -> (logical OR=w308:bool)
            n178 = case shown="True" w308 {
              tunnel: w307 -> [_ w323]
              frame False {
              }
              frame True {
                n179 = One Button Dialog(message=w323) -> ()  [unwired: 1 in, 1 out]
              }
            }
          }
        }
      }
    }
    frame Error {
    }
  }
